vi "scanchannel_no_setting.vi"(0 "Instrument VISA in":T1={"AWG VISA"="81160A", "Oscilloscope  VISA "="labosc4", "Integration Board IP"="172.16.7.43", "connection ID"=refnum, "report out"=refnum, "report file path"=path "D:/CTA/Data_test/test3a"}, 5 "error in":errorcluster, 7 "L1 Address":i32=17, 9 "Ch burst":i32=10000, 13 "initial value":i32=50) -> (8 "XY Graph":cluster{"Y":dbl[], "Y":dbl[]}[](graph), 10 "XY Graph 2":cluster{"Y":dbl[], "Y":dbl[]}[](graph), 12 "appended array":dbl[](array[numeric]), 14 "output cluster":T1, 15 "L1 value":i32, 19 "error out":errorcluster)   [LabVIEW 2009]
uses:
  <vilib>/Utility/NIReport.llb/NI_report.lvclass
  <vilib>/Utility/NIReport.llb/HTML/NI_HTML.lvclass
  <vilib>/Analysis/NI_AALPro.lvlib
  <instrlib>/Agilent 8000 Series/Agilent 8000 Series.lvlib
  <instrlib>/Agilent 81150/Agilent 81150.lvlib
panel:
  out "Pulse Error":dbl caption="Measurement"
  out "Amp Error":dbl caption="Measurement"
  out "Pulse with":dbl caption="Measurement"
  out "Amplitude":dbl caption="Measurement"
  out "concatenated string":string
  out "IPR value":i32
  out "Numeric":i32
  out "Data out":string="ACK\r\n"
  out "x .and. y?":bool
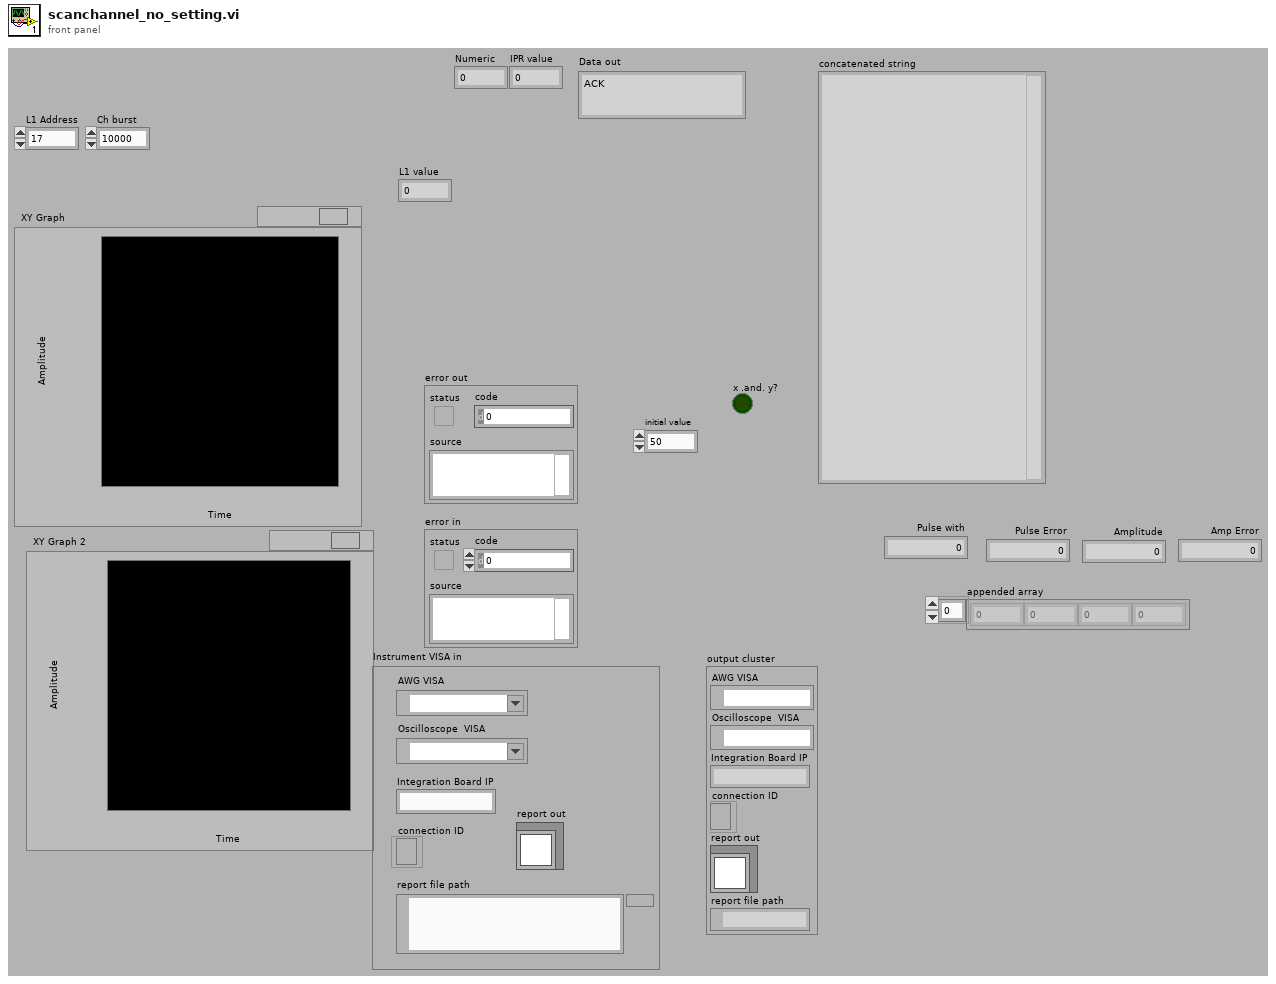
[diagram p1: front panel]
types:
  T1 = cluster{"AWG VISA":refnum<visa-resource-name>, "Oscilloscope  VISA ":refnum<visa-resource-name>, "Integration Board IP":string, "connection ID":refnum<k5>, "report out":refnum<class "NI_report.lvclass">, "report file path":path}
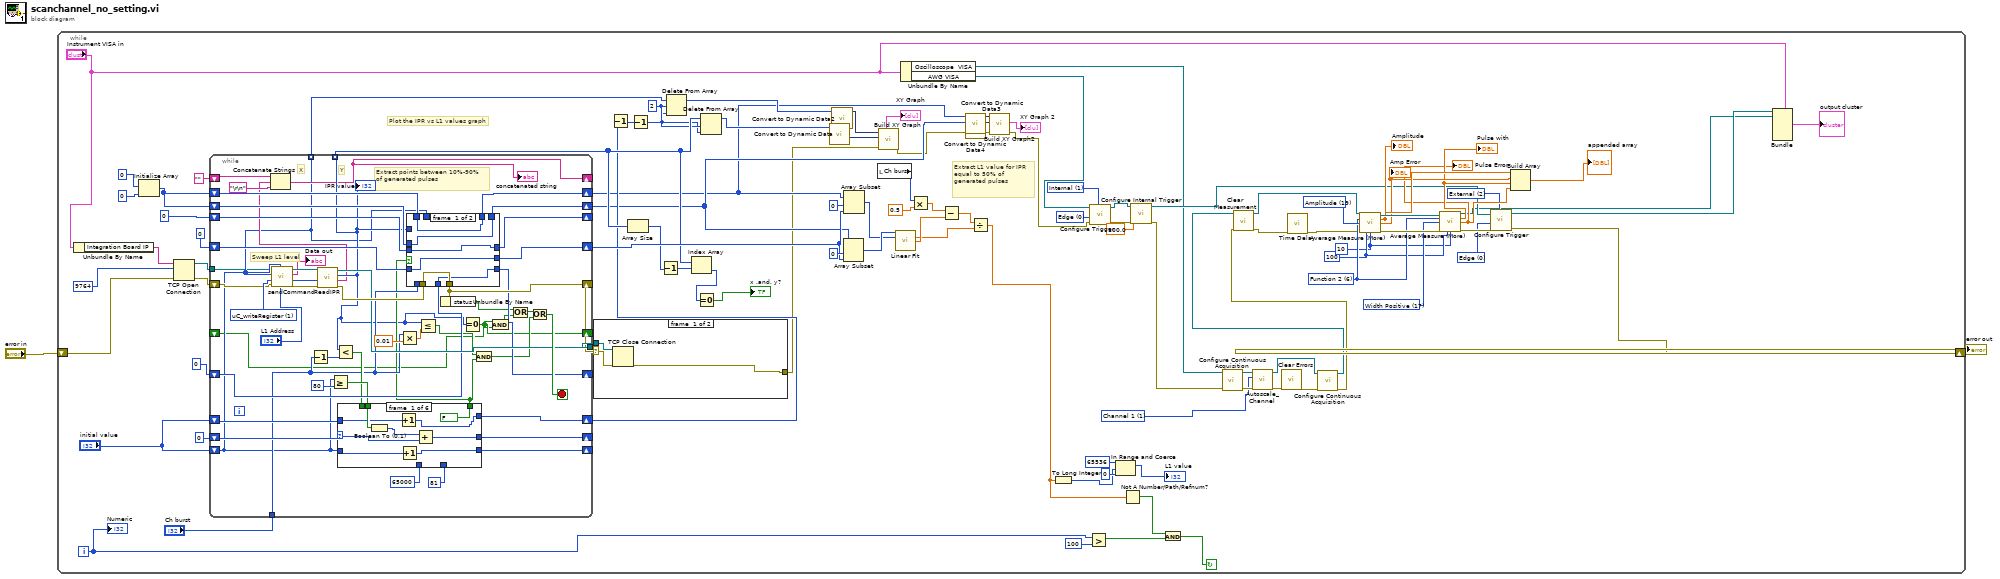
[diagram p0: block diagram]
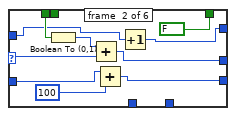
[diagram p2: hidden frame]
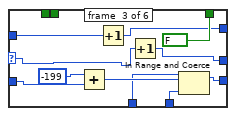
[diagram p3: hidden frame]
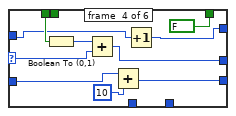
[diagram p4: hidden frame]
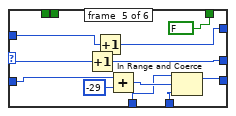
[diagram p5: hidden frame]
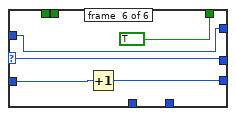
[diagram p6: hidden frame]
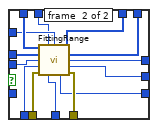
[diagram p7: hidden frame]
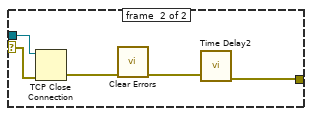
[diagram p8: hidden frame]
diagram:
  n1 = while {
    shift-right: [w21] -> w2
    shift-left: "error in" -> [w47]
    i -> [w50]
    stop <- w51 continue-if-true
    w17 = 1 items=["Channel 1"=1, "Channel 2"=2, "Channel 3"=3, "Channel 4"=4, "Function 1"=5, "Function 2"=6, "Function 3"=7, "Function 4"=8, "Memory 1"=9, "Memory 2"=10, "Memory 3"=11, "Memory 4"=12] ("Channel")
    w27 = u16 2 items=["Immediate", "Internal", "External", "Software Trigger Function"] ("Trigger Source (0: Immediate)")
    w28 = u16 0 items=["Edge", "Level"] ("Trigger Mode (0: Edge)")
    w35 = u32 10 ("Max Errors")
    w36 = u32 100 ("Averages")
    w37 = 17 items=["Rise Time", "Fall Time", "Frequency", "Period", "Voltage RMS(AC)", "Voltage RMS(DC)", "Voltage RMS (AC,cycle)", "Voltage RMS (DC,cycle)", "Voltage Max", "Voltage Min", "Voltage Middle", "Voltage Vpp", "Voltage High", "Voltage Low", "Voltage Average", "Voltage Average (cycle)", "Width Negative", "Width Positive", "Duty Cycle Positive", "Amplitude", "Overshoot", "Preshoot", "Voltage Base", "Voltage Upper", "Time Max", "Time Min", "Color Grade Crossing", "Color Grade Eye Width", "Color Grade Eye Height", "Color Grade Eye Q-Factory", "Color Grade Eye Duty Cycle Distortion(Percent)", "Color Grade Eye Duty Cycle Distortion(Time)", "Color Grade Eye Jitter(PP)", "Color Grade Eye Width(RMS)", "Cycle-cycle Duty Jitter(Rising)", "Cycle-cycle Duty Jitter(Falling)", "Cycle-cycle Jitter(Rising)", "Cycle-cycle Jitter(Falling)", "Cycle-cycle - Width", "Cycle-cycle + Width", "Date Rate", "Unit Interval", "FFT Delta Frequency", "FFT Delta Magnitude", "FFT Frequency", "FFT Magnitude", "Slew Rate", "Area (Entire Display)", "Area(Single Cycle)", "Duty Cycle (Rising)", "Duty Cycle (Falling)"] ("Measurement Function (0: Rise Time)")
    w41 = 19 items=["Rise Time", "Fall Time", "Frequency", "Period", "Voltage RMS(AC)", "Voltage RMS(DC)", "Voltage RMS (AC,cycle)", "Voltage RMS (DC,cycle)", "Voltage Max", "Voltage Min", "Voltage Middle", "Voltage Vpp", "Voltage High", "Voltage Low", "Voltage Average", "Voltage Average (cycle)", "Width Negative", "Width Positive", "Duty Cycle Positive", "Amplitude", "Overshoot", "Preshoot", "Voltage Base", "Voltage Upper", "Time Max", "Time Min", "Color Grade Crossing", "Color Grade Eye Width", "Color Grade Eye Height", "Color Grade Eye Q-Factory", "Color Grade Eye Duty Cycle Distortion(Percent)", "Color Grade Eye Duty Cycle Distortion(Time)", "Color Grade Eye Jitter(PP)", "Color Grade Eye Width(RMS)", "Cycle-cycle Duty Jitter(Rising)", "Cycle-cycle Duty Jitter(Falling)", "Cycle-cycle Jitter(Rising)", "Cycle-cycle Jitter(Falling)", "Cycle-cycle - Width", "Cycle-cycle + Width", "Date Rate", "Unit Interval", "FFT Delta Frequency", "FFT Delta Magnitude", "FFT Frequency", "FFT Magnitude", "Slew Rate", "Area (Entire Display)", "Area(Single Cycle)", "Duty Cycle (Rising)", "Duty Cycle (Falling)"] ("Measurement Function (0: Rise Time)")
    w38 = 6 items=["Channel 1"=1, "Channel 2"=2, "Channel 3"=3, "Channel 4"=4, "Function 1"=5, "Function 2"=6, "Function 3"=7, "Function 4"=8, "Memory 1"=9, "Memory 2"=10, "Memory 3"=11, "Memory 4"=12] ("Channel (1: Channel 1)")
    w43 = u16 0 items=["Edge", "Level"] ("Trigger Mode (0: Edge)")
    w44 = u16 1 items=["Immediate", "Internal", "External", "Software Trigger Function"] ("Trigger Source (0: Immediate)")
    w80 = 2 ("length")
    # "Extract L1 value for IPR equal to 50% of generated pulses"
    # "Plot the IPR vs L1 values graph"
    n2 = Unbundle By Name("Instrument VISA in") -> ("Integration Board IP"=w15:string)
    n3 = Initialize Array(0 ("element"), 0 ("dimension size")) -> (w68:i32[])
    n4 = TCP Open Connection(address=w15, remote port or service name=u16 9764, error in (no error)=w47) -> (connection ID=w46:refnum<k5>, error out=w45:errorcluster)  [unwired: 2 in]
    n5 = while {
      tunnel: [w118] -> w83 mode=indexing
      tunnel: [w111] -> w85 mode=indexing
      shift-right: [w151] -> w72
      shift-left: w68 -> [w149]
      shift-right: [w150] -> w76
      shift-left: w68 -> [w148]
      shift-right: [w144] -> w54
      shift-left: w45 -> [w136]
      shift-right: [w146] -> _
      shift-left: 0 ("Array Pointer out") -> [w147]
      tunnel: [w137] -> w60
      shift-right: [w145] -> w94
      shift-left: 0 ("N_Array Elements") -> [w135]
      shift-right: [w133] -> _
      shift-left: 0 ("State machine") -> [w134]
      tunnel: "Ch burst" -> [w123]
      shift-right: [w129] -> _
      shift-left: 0 -> [w131]
      shift-right: [w128] -> _
      shift-left: "initial value" -> [w111]
      shift-right: [w126] -> w81
      shift-left: "initial value" -> [w125]
      shift-right: [w115] -> _
      shift-left: "" -> [w116]
      shift-right: [w108] -> _
      shift-left: _ -> [w107]
      tunnel: w46 -> [w104]
      stop <- w143 stop-if-true
      w142 = u16 1 items=["sendCommand"=9, "FPGA_writeRegister"=3, "FPGA_readRegister"=2, "uC_writeRegister"=1, "uC_readRegister"=0] ("Action")
      # "Extract points between 10%-90% of generated pulses"
      # "Sweep L1 level"
      # "Y"
      # "X"
      n6 = call "sendCommand.vi"("Address"="L1 Address", "Data"=w111, "error in"=w136, "Action"=w142, "id_in"=w111, "connection ID"=w104) -> ("error out"=w141:errorcluster, "id_out"=w114:i32, "Data out"=→"Data out":string, "connection ID out"=w140:refnum<k5>)  [unwired: 1 in, 1 out]
      n7 = Decrement(x=w123) -> (x-1=w124:i32)
      n8 = call "ReadIPR.vi"("error in"=w141, "id_in"=w114, "connection ID"=w140) -> ("error out"=w139:errorcluster, "Data out"=w112:string, "IPR value"=w118:i32, "connection ID out"=w137:refnum<k5>)  [unwired: 4 in, 1 out]
      "IPR value" <- w118
      n9 = Concatenate Strings(w116, w112, "\r\n") -> (w115:string)
      "concatenated string" <- w115
      n10 = Greater Or Equal?(x=w111, y=80) -> (x >= y?=w130:bool)
      n11 = Less?(x=w118, y=w124) -> (x < y?=w127:bool)
      n12 = case shown="0, Default" w131 {
        selector: w131 -> [w160 w170 w183 w188 w201 w207]
        tunnel: w130 -> [w162 _ _ _ _ _]
        tunnel: [w159 w169 w179 w186 w200 w207] -> w129
        tunnel: [w157 w166 w175 w191 w196 w208] -> w128
        tunnel: w111 -> [w158 w168 w182 w192 w203 w209]
        tunnel: w127 -> [_ w172 _ w189 _ _]
        tunnel: [FALSE FALSE FALSE FALSE FALSE TRUE] -> w122
        tunnel: [w155 w164 w178 w185 w199 w205] -> w126
        tunnel: w125 -> [w154 w163 w177 w184 w202 w205]
        tunnel: 81 ("lower limit") -> [_ _ w174 _ w195 _]
        tunnel: 65000 ("upper limit") -> [_ _ w173 _ w194 _]
        frame #0 {
          n13 = Boolean To (0,1)(Boolean=w162) -> (0, 1=w161:i16)
          n14 = Increment(x=w154) -> (x+1=w155:i32)
          n15 = Increment(x=w158) -> (x+1=w157:i32)
          n16 = Add(x=w161, y=w160) -> (x+y=w159:i32)
        }
        frame #1 {
          n17 = Boolean To (0,1)(Boolean=w172) -> (0, 1=w171:i16)
          n18 = Add(x=w171, y=w170) -> (x+y=w169:i32)
          n19 = Add(x=w168, y=100) -> (x+y=w166:i32)
          n20 = Increment(x=w163) -> (x+1=w164:i32)
        }
        frame #2 {
          n21 = Add(x=-199, y=w182) -> (x+y=w176:i32)
          n22 = Increment(x=w177) -> (x+1=w178:i32)
          n23 = Increment(x=w183) -> (x+1=w179:i32)
          n24 = In Range and Coerce(upper limit=w173, x=w176, lower limit=w174) -> (coerced(x)=w175:i32)  [unwired: 1 out]
        }
        frame #3 {
          n25 = Boolean To (0,1)(Boolean=w189) -> (0, 1=w187:i16)
          n26 = Add(x=w187, y=w188) -> (x+y=w186:i32)
          n27 = Add(x=w192, y=10) -> (x+y=w191:i32)
          n28 = Increment(x=w184) -> (x+1=w185:i32)
        }
        frame #4 {
          n29 = Increment(x=w201) -> (x+1=w200:i32)
          n30 = Increment(x=w202) -> (x+1=w199:i32)
          n31 = Add(x=w203, y=-29 ("x")) -> (x+y=w197:i32)
          n32 = In Range and Coerce(upper limit=w194, x=w197, lower limit=w195) -> (coerced(x)=w196:i32)  [unwired: 1 out]
        }
        frame #5 {
          n33 = Increment(x=w209) -> (x+1=w208:i32)
        }
      }
      n34 = Multiply(x=w123, y=0.01) -> (x*y=w152:dbl)
      n35 = case shown="False" w122 {
        tunnel: [w215 w229] -> w151
        tunnel: [w214 w228] -> w150
        tunnel: w149 -> [w215 w227]
        tunnel: w148 -> [w214 w226]
        tunnel: w147 -> [w212 w225]
        tunnel: [w212 w224] -> w146
        tunnel: [w211 w223] -> w145
        tunnel: w123 -> [_ w222]
        tunnel: [w213 w221] -> w144
        tunnel: w139 -> [w213 w220]
        tunnel: w118 -> [_ w219]
        tunnel: w111 -> [_ w218]
        tunnel: w135 -> [w211 _]
        tunnel: w134 -> [w210 w217]
        tunnel: [w210 w216] -> w133
        frame #0 {
        }
        frame #1 {
          n36 = call "FittingRange.vi"("Array in (X)"=w227, "L0 DAC"=w218, "IPR"=w219, "Array in (Y)"=w226, "Array Pointer in"=w225, "Cycles Burst"=w222, "error in"=w220, "State machine"=w217) -> ("Array out (X)"=w229:i32[], "Array out (Y)"=w228:i32[], "Array Pointer out"=w224:i32, "N_Array Elements"=w223:i32, "State machine"=w216:i32, "error out"=w221:errorcluster)  [unwired: 2 in]
        }
      }
      n37 = Less Or Equal?(x=w118, y=w152) -> (x <= y?=w121:bool)
      n38 = Unbundle By Name(w144) -> ("status"=w119:bool)
      n39 = Equal To 0?(x=w118) -> (x = 0?=w108:bool)
      n40 = And(x=w121, y=w122) -> (x .and. y?=w120:bool)
      n41 = And(x=w108, y=w107) -> (x .and. y?=w109:bool)
      n42 = Or(x=w119, y=w109) -> (x .or. y?=w110:bool)
      n43 = Or(x=w110, y=w120) -> (x .or. y?=w143:bool)
    }
    n44 = case shown="Error" w54 {
      selector: w54 -> [w231 w236]
      tunnel: w60 -> [w232 w237]
      tunnel: [w230 w235] -> w58
      frame #0 {
        n45 = TCP Close Connection(connection ID=w232, error in (no error)=w231) -> (error out=w230:errorcluster)  [unwired: 1 in, 1 out]
      }
      frame #1 {
        n46 = TCP Close Connection(connection ID=w237, error in (no error)=w236) -> (error out=w234:errorcluster)  [unwired: 1 in, 1 out]
        n47 = call <vilib>:"Clear Errors.vi"("error in (no error)"=w234) -> ("error out"=w233:errorcluster)  [unwired: 6 in]
        n48 = call "Time Delay2"("error in (no error)"=w233) -> ("error out"=w235:errorcluster)  [unwired: 10 in]
      }
    }
    n49 = Decrement(x=w81) -> (x-1=w78:i32)
    n50 = Array Size(array=w83) -> (size(s)=w63:i32)
    n51 = Decrement(x=w78) -> (x-1=w79:i32)
    n52 = Decrement(x=w63) -> (x-1=w64:i32)
    n53 = Delete From Array(array=w85, length=w80, index=w79) -> (array with subset deleted=w84:i32[])  [unwired: 1 out]
    n54 = Index Array(array=w83, index=w64) -> (element=w61:i32)
    n55 = Equal To 0?(x=w61) -> (x = 0?=→"x .and. y?":bool)
    n56 = Delete From Array(array=w83, length=w80, index=w79) -> (array with subset deleted=w82:i32[])  [unwired: 1 out]
    n57 = call "Convert to Dynamic Data"("Array"=w82) -> ("Dynamic Data Type"=w98:dynamicdata)  [unwired: 3 in]
    n58 = call "Convert to Dynamic Data2"("Array"=w84) -> ("Dynamic Data Type"=w97:dynamicdata)  [unwired: 3 in]
    n59 = Array Subset(array=w76, index=0, length=w94) -> (w93:i32[])
    n60 = Array Subset(array=w72, index=0, length=w94) -> (w92:i32[])
    n61 = local read "Ch burst"() -> (w86:i32)
    n62 = call "Build XY Graph"("error in (no error)"=w58, "Y Input"=w98, "X Input"=w97) -> ("error out"=w74:errorcluster, "XY Graph"=→"XY Graph":cluster{"Y":dbl[], "Y":dbl[]}[])  [unwired: 7 in]
    n63 = call <vilib>:"Linear Fit.vi"("Y"=w93, "X"=w92) -> ("slope"=w87:dbl, "intercept"=w89:dbl)  [unwired: 9 in, 3 out]
    n64 = Unbundle By Name("Instrument VISA in") -> ("Oscilloscope  VISA"=w13:refnum<visa-resource-name>, "AWG VISA"=w14:refnum<visa-resource-name>)
    n65 = Multiply(x=w86, y=0.5) -> (x*y=w90:dbl)
    n66 = Subtract(x=w90, y=w89) -> (x-y=w88:dbl)
    n67 = call "Convert to Dynamic Data3"("Array"=w72) -> ("Dynamic Data Type"=w77:dynamicdata)  [unwired: 3 in]
    n68 = call "Convert to Dynamic Data4"("Array"=w76) -> ("Dynamic Data Type"=w75:dynamicdata)  [unwired: 3 in]
    n69 = Divide(x=w88, y=w87) -> (x/y=w56:dbl)
    n70 = call "Build XY Graph2"("error in (no error)"=w74, "Y Input"=w75, "X Input"=w77) -> ("error out"=w22:errorcluster, "XY Graph"=→"XY Graph 2":cluster{"Y":dbl[], "Y":dbl[]}[])  [unwired: 7 in]
    n71 = To Long Integer(number=w56) -> (32bit integer=w100:i32)
    n72 = Greater?(x=w50, y=100) -> (0:w53:bool)
    n73 = call <instrlib>:"Configure Trigger.vi"("Trigger Source (0: Immediate)"=w44, "error in (no error)"=w22, "Trigger Mode (0: Edge)"=w43, "VISA resource name"=w14) -> ("error out"=w26:errorcluster, "VISA resource name out"=w24:refnum<visa-resource-name>)  [unwired: 6 in]
    n74 = In Range and Coerce(upper limit=65536, x=w100, lower limit=0) -> (coerced(x)=→"L1 value":i32)  [unwired: 1 out]
    n75 = Not A Number/Path/Refnum?(number/path/refnum=w56) -> (NaN/Path/Refnum?=w52:bool)
    n76 = call <instrlib>:"Configure Internal Trigger.vi"("error in (no error)"=w26, "Frequency (100000.0 Hz)"=100.0, "VISA resource name"=w24) -> ("error out"=w16:errorcluster, "VISA resource name out"=w25:refnum<visa-resource-name>)  [unwired: 7 in]
    n77 = And(x=w52, y=w53) -> (x .and. y?=w51:bool)
    n78 = call <instrlib>:"Configure Continuous Acquisition.vi"("error in (no error)"=w16, "VISA resource name"=w13) -> ("error out"=w20:errorcluster, "VISA resource name out"=w18:refnum<visa-resource-name>)  [unwired: 8 in]
    n79 = call "Autoscale_Channel.vi"("error in"=w20, "Channel"=w17, "VISA resource name"=w18) -> ("error out"=w19:errorcluster, "VISA resource name out"=w7:refnum<visa-resource-name>)  [unwired: 5 in, 2 out]
    n80 = call <vilib>:"Clear Errors.vi"("error in (no error)"=w19) -> ("error out"=w8:errorcluster)  [unwired: 6 in]
    n81 = call <instrlib>:"Configure Continuous Acquisition.vi"("error in (no error)"=w8, "VISA resource name"=w7) -> ("error out"=w5:errorcluster, "VISA resource name out"=w6:refnum<visa-resource-name>)  [unwired: 8 in]
    n82 = call <instrlib>:"Clear Measurement.vi"("error in (no error)"=w5, "VISA resource name"=w6) -> ("error out"=w4:errorcluster, "VISA resource name out"=w42:refnum<visa-resource-name>)  [unwired: 8 in]
    n83 = call "Time Delay"("error in (no error)"=w4) -> ("error out"=w3:errorcluster)  [unwired: 10 in]
    n84 = call "Average Measure (More).vi"("VISA resource name"=w42, "Channel (1: Channel 1)"=w38, "Measurement Function (0: Rise Time)"=w41, "error in (no error)"=w3, "Averages"=w36, "Max Errors"=w35) -> ("VISA resource name out"=w40:refnum<visa-resource-name>, "Measure Average"=w34:dbl, "Measure Error"=w33:dbl, "error out"=w39:errorcluster)  [unwired: 6 in]
    "Amplitude" <- w34
    "Amp Error" <- w33
    n85 = call "Average Measure (More).vi"("VISA resource name"=w40, "Channel (1: Channel 1)"=w38, "Measurement Function (0: Rise Time)"=w37, "error in (no error)"=w39, "Averages"=w36, "Max Errors"=w35) -> ("VISA resource name out"=w10:refnum<visa-resource-name>, "Measure Average"=w32:dbl, "Measure Error"=w31:dbl, "error out"=w29:errorcluster)  [unwired: 6 in]
    "Pulse with" <- w32
    "Pulse Error" <- w31
    n86 = call <instrlib>:"Configure Trigger.vi"("Trigger Source (0: Immediate)"=w27, "error in (no error)"=w29, "Trigger Mode (0: Edge)"=w28, "VISA resource name"=w25) -> ("error out"=w21:errorcluster, "VISA resource name out"=w11:refnum<visa-resource-name>)  [unwired: 6 in]
    n87 = Build Array(w34, w33, w32, w31) -> (→"appended array":dbl[])
    n88 = Bundle(cluster="Instrument VISA in", "AWG VISA"=w11, "Oscilloscope  VISA"=w10) -> (→"output cluster":T1)  [unwired: 4 in]
    "Numeric" <- w50
  }
  "error out" <- w2
